vi "subCheckForShallowDependencyProcessing.vi"(6 "Shallow deps?":bool, 9 "ILabVIEWItem to enqueue":refnum<class "ILabVIEWItem.lvclass">, 11 "Current ILabVIEWItem in":refnum<class "ILabVIEWItem.lvclass">) -> (1 "Process?":bool, 3 "Current ILabVIEWItem":refnum<class "ILabVIEWItem.lvclass">)   [LabVIEW 2020, in "DependencyInspection.lvlib" / "CDependencyList.lvclass"]
uses:
  CDependencyList.lvclass
  LabVIEWObjectInterfaces/ILabVIEWItem/ILabVIEWItem.lvclass
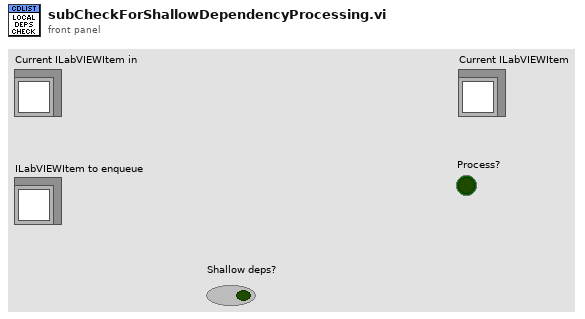
[diagram p1: front panel]
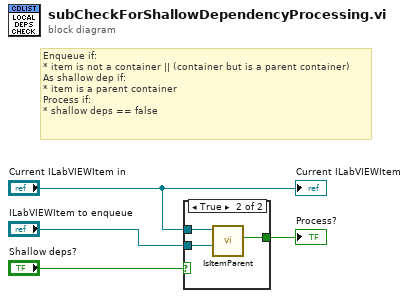
[diagram p0: block diagram]
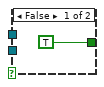
[diagram p2: hidden frame]
diagram:
  # "Enqueue if:\n* item is not a container || (container but is a parent container)\nAs shallow dep if:\n* item is a parent container\nProcess if:\n* shallow deps == false"
  n1 = case shown="True" "Shallow deps?" {
    tunnel: "Current ILabVIEWItem in" -> [_ w8]
    tunnel: "ILabVIEWItem to enqueue" -> [_ w7]
    tunnel: [TRUE ("Is parent?") w6] -> w3
    frame False {
    }
    frame True {
      n2 = call-dynamic "IsItemParent.vi"("Item to compare"=w7, "ILabVIEWItem in"=w8) -> ("Is parent?"=w6:bool)  [unwired: 7 in, 2 out]
    }
  }
  "Process?" <- w3
  "Current ILabVIEWItem" <- "Current ILabVIEWItem in"
